vi "Shrink ROI.vi"(7 "ROI Change":enum16{"Extend", "Shrink"}(ring)=enum."Shrink", 8 "error in (no error)":errorcluster, 11 "ROI in":T2) -> (0 "error out":errorcluster, 3 "ROI Descriptor":T1 {"Contours"."Type" items=["No Selection", "Point", "Line", "Rectangle", "Oval", "Polygon", "Freehand Region", "Annulus", "Unused2", "Unused3", "Broken Line", "Freehand Line", "Rotated Rectangle"]})   [LabVIEW 2020]
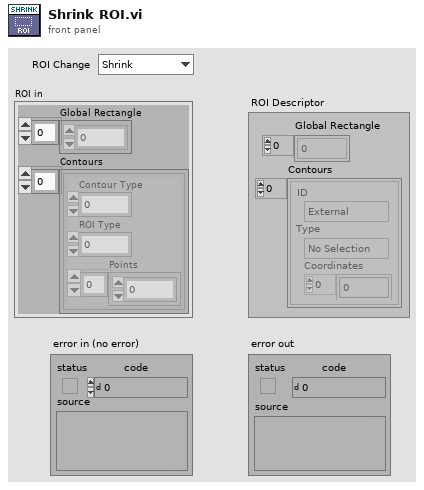
[diagram p1: front panel]
types:
  T1 = typedef "ROI Descriptor" = cluster{"Global Rectangle":i32[], "Contours":cluster{"ID":enum32{"External", "Internal"}, "Type":u32, "Coordinates":i32[]}[]}
  T2 = cluster{"Global Rectangle":i32[], "Contours":cluster{"Contour Type":u32, "ROI Type":u32, "Points":i32[]}[]}
  T3 = cluster{"Contour Type":u32, "ROI Type":u32, "Points":i32[]}[]
  T4 = cluster{"Contour Type":u32, "ROI Type":u32, "Points":i32[]}
  T5 = typedef "IMAQ Rectangle" = cluster{"Left":i32, "Top":i32, "Right":i32, "Bottom":i32, "Rotation":dbl}
  T6 = cluster{"ID":enum32{"External", "Internal"}, "Type":u32, "Coordinates":i32[]}[]
  T7 = cluster{"ID":enum32{"External", "Internal"}, "Type":u32, "Coordinates":i32[]}
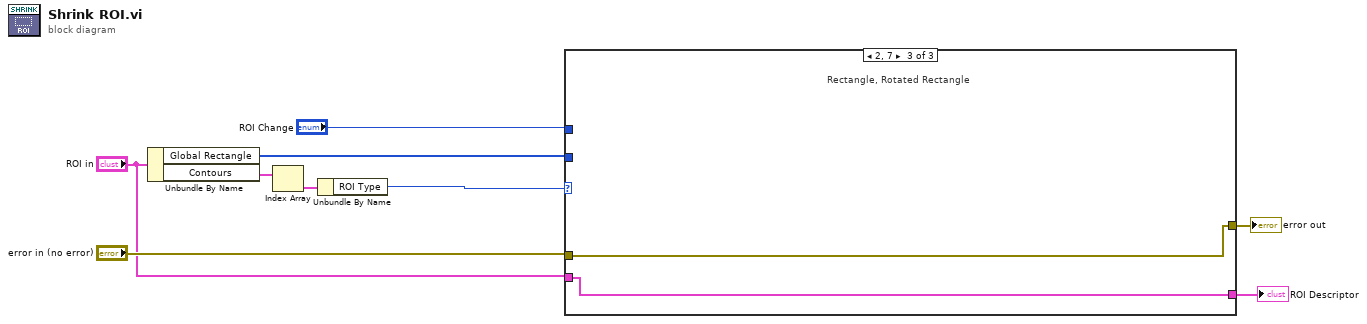
[diagram p0: block diagram]
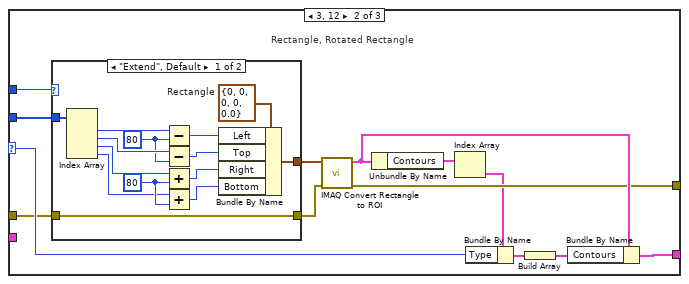
[diagram p3: hidden frame]
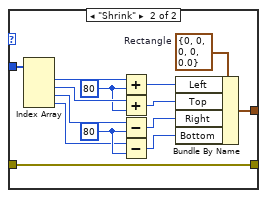
[diagram p4: hidden frame]
diagram:
  n1 = Unbundle By Name("ROI in") -> ("Global Rectangle"=w9:i32[], "Contours"=w6:T3)
  n2 = Index Array(array=w6) -> (element=w3:T4)  [unwired: 1 in]
  n3 = Unbundle By Name(w3) -> ("ROI Type"=w5:u32)
  n4 = case shown="2, 7" w5 {
    selector: w5 -> [_ w21 _]
    tunnel: w9 -> [_ w24 _]
    tunnel: [w11 w17 w54] -> w2
    tunnel: "error in (no error)" -> [w10 w14 w53]
    tunnel: [w10 w16 w53] -> w7
    tunnel: "ROI in" -> [w11 _ w54]
    tunnel: "ROI Change" -> [_ w12 _]
    frame 0, Default {
    }
    frame 3, 12 {
      # "Rectangle, Rotated Rectangle"
      n5 = case shown="\"Extend\", Default" w12 {
        tunnel: w24 -> [w38 w52]
        tunnel: [w26 w40] -> w23
        tunnel: w14 -> [w25 w39]
        tunnel: [w25 w39] -> w13
        frame "Extend", Default {
          w31 = T5 {"Left"=0, "Top"=0, "Right"=0, "Bottom"=0, "Rotation"=0.0}  # Rectangle
          w34 = 80
          w35 = 80
          n6 = Index Array(array=w38) -> (element #1=w37:i32, element #2=w36:i32, element #3=w33:i32, element #4=w32:i32)  [unwired: 4 in]
          n7 = Subtract(x=w37, y=w35) -> (x-y=w30:i32)
          n8 = Subtract(x=w36, y=w35) -> (x-y=w29:i32)
          n9 = Add(x=w33, y=w34) -> (x+y=w28:i32)
          n10 = Add(x=w32, y=w34) -> (x+y=w27:i32)
          n11 = Bundle By Name(cluster=w31, "Left"=w30, "Top"=w29, "Right"=w28, "Bottom"=w27) -> (w26:T5)
        }
        frame "Shrink" {
          w45 = T5 {"Left"=0, "Top"=0, "Right"=0, "Bottom"=0, "Rotation"=0.0}  # Rectangle
          w48 = 80
          w49 = 80
          n12 = Index Array(array=w52) -> (element #1=w51:i32, element #2=w50:i32, element #3=w47:i32, element #4=w46:i32)  [unwired: 4 in]
          n13 = Add(x=w51, y=w49) -> (x+y=w44:i32)
          n14 = Add(x=w50, y=w49) -> (x+y=w43:i32)
          n15 = Subtract(x=w47, y=w48) -> (x-y=w42:i32)
          n16 = Subtract(x=w46, y=w48) -> (x-y=w41:i32)
          n17 = Bundle By Name(cluster=w45, "Left"=w44, "Top"=w43, "Right"=w42, "Bottom"=w41) -> (w40:T5)
        }
      }
      n18 = call "IMAQ Convert Rectangle to ROI"("error in (no error)"=w13, "Rectangle"=w23) -> ("error out"=w16:errorcluster, "ROI Descriptor"=w20:T1)  [unwired: 7 in]
      n19 = Unbundle By Name(w20) -> ("Contours"=w22:T6)
      n20 = Index Array(array=w22) -> (element=w15:T7)  [unwired: 1 in]
      n21 = Bundle By Name(cluster=w15, "Type"=w21) -> (w19:T7)
      n22 = Build Array(w19) -> (w18:T6)
      n23 = Bundle By Name(cluster=w20, "Contours"=w18) -> (w17:T1)
    }
    frame 2, 7 {
      # "Rectangle, Rotated Rectangle"
    }
  }
  "error out" <- w7
  "ROI Descriptor" <- w2
